vi "ChildControlsInCluster.vi"(8 "error in (no error)":errorcluster, 11 "Control in":refnum<vi>) -> (0 "error out":errorcluster, 2 "IsCluster":bool, 3 "Controls[]":refnum<vi>[](array[refnum]))   [LabVIEW 2021, in "SetGetControlValue.lvlib"]
uses:
  SetGetControlValue.lvlib
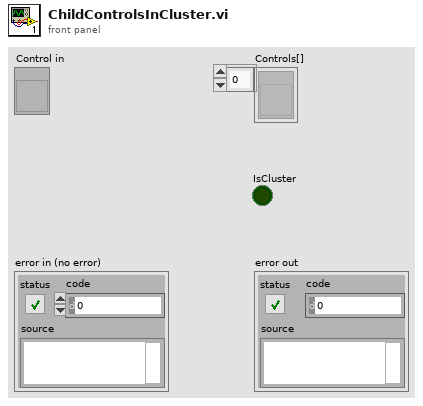
[diagram p1: front panel]
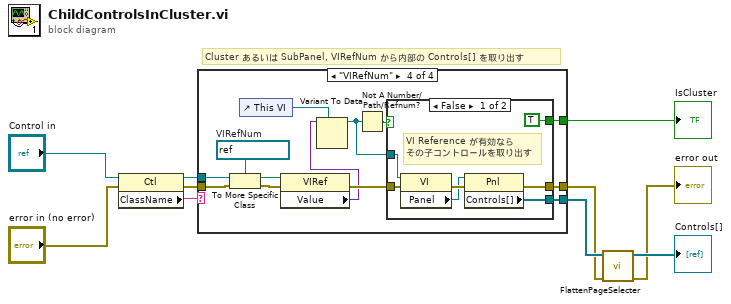
[diagram p0: block diagram]
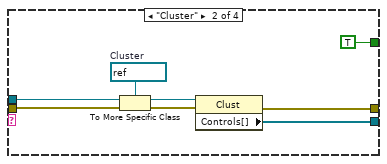
[diagram p3: hidden frame]
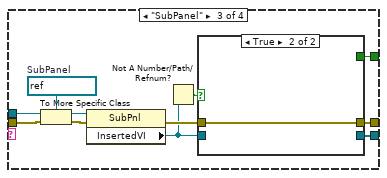
[diagram p4: hidden frame]
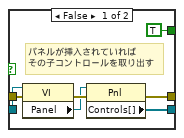
[diagram p5: hidden frame]
diagram:
  # "Cluster あるいは SubPanel, VIRefNum から内部の Controls[] を取り出す"
  n1 = property class="Ctl"(reference="Control in", error in="error in (no error)") -> (reference out=w4:refnum<vi>, error out=w5:errorcluster, "ClassName"=w8:string)
  n2 = case shown="\"VIRefNum\"" w8 {
    tunnel: [_ w17 w25 w46] -> w10
    tunnel: [_ TRUE w23 w44] -> w7
    tunnel: w5 -> [w11 w15 w27 w48]
    tunnel: [w11 w13 w24 w45] -> w2
    tunnel: w4 -> [_ w12 w22 w43]
    frame Default {
    }
    frame "Cluster" {
      w19 = refnum<vi> refnum  # Cluster
      n3 = To More Specific Class(target class=w19, reference=w12, error in=w15) -> (specific class reference=w18:refnum<vi>, error out=w14:errorcluster)
      n4 = property class="Clust"(reference=w18, error in=w14) -> (error out=w13:errorcluster, "Controls[]"=w17:refnum<vi>[])  [unwired: 1 out]
    }
    frame "SubPanel" {
      w30 = refnum<vi> refnum  # SubPanel
      n5 = To More Specific Class(target class=w30, reference=w22, error in=w27) -> (specific class reference=w29:refnum<vi>, error out=w28:errorcluster)
      n6 = property class="SubPnl"(reference=w29, error in=w28) -> (error out=w26:errorcluster, "InsertedVI"=w21:refnum<vi>)  [unwired: 1 out]
      n7 = Not A Number/Path/Refnum?(number/path/refnum=w21) -> (NaN/Path/Refnum?=w20:bool)
      n8 = case shown="True" w20 {
        tunnel: w21 -> [w37 _]
        tunnel: w26 -> [w36 w38]
        tunnel: [w33 _] -> w25
        tunnel: [w32 w38] -> w24
        tunnel: [TRUE _] -> w23
        frame False {
          # "パネルが挿入されていれば\nその子コントロールを取り出す"
          n9 = property class="VI"(reference=w37, error in=w36) -> (error out=w35:errorcluster, "Panel"=w34:refnum<vi>)  [unwired: 1 out]
          n10 = property class="Pnl"(reference=w34, error in=w35) -> (error out=w32:errorcluster, "Controls[]"=w33:refnum<vi>[])  [unwired: 1 out]
        }
        frame True {
        }
      }
    }
    frame "VIRefNum" {
      w51 = refnum<vi> refnum  # VIRefNum
      n11 = To More Specific Class(target class=w51, reference=w43, error in=w48) -> (specific class reference=w50:refnum<vi>, error out=w49:errorcluster)
      n12 = control-ref of="This VI"() -> (w41:refnum<vi>)
      n13 = property class="VIRef"(reference=w50, error in=w49) -> (error out=w47:errorcluster, "Value"=w40:variant)  [unwired: 1 out]
      n14 = Variant To Data(type=w41, Variant=w40) -> (data=w39:refnum<vi>)  [unwired: 1 in, 1 out]
      n15 = Not A Number/Path/Refnum?(number/path/refnum=w39) -> (NaN/Path/Refnum?=w42:bool)
      n16 = case shown="False" w42 {
        tunnel: w39 -> [w58 _]
        tunnel: w47 -> [w57 w59]
        tunnel: [w54 _] -> w46
        tunnel: [w53 w59] -> w45
        tunnel: [TRUE _] -> w44
        frame False {
          # "VI Reference が有効なら\nその子コントロールを取り出す"
          n17 = property class="VI"(reference=w58, error in=w57) -> (error out=w56:errorcluster, "Panel"=w55:refnum<vi>)  [unwired: 1 out]
          n18 = property class="Pnl"(reference=w55, error in=w56) -> (error out=w53:errorcluster, "Controls[]"=w54:refnum<vi>[])  [unwired: 1 out]
        }
        frame True {
        }
      }
    }
  }
  "IsCluster" <- w7
  n19 = call "FlattenPageSelecter.vi"("error in (no error)"=w2, "Controls[]"=w10) -> ("error out"=→"error out":errorcluster, "Flatten[]"=→"Controls[]":refnum<vi>[])  [unwired: 8 in]
